vi "Vision Research Phantom Series PhFile PhNewCineFromCamera.vi"(0 "Camera Number in":u32=1, 1 "CineNr in":i32=1, 5 "Error In (no error)":errorcluster) -> (14 "Camera Number out":u32=1, 15 "CineNr out":i32, 17 "pCH":u64, 19 "Error Out":errorcluster)   [LabVIEW 2013, in "VRI.lvlib"]
doc: "PhFile.dll\n\nPhNewCineFromCamera\nHRESULT PhNewCineFromCamera(INT CN, INT CineNr, PCINEHANDLE pCH);\n\nParameters Description\nCN(in) Camera number.\nCineNr(in) Cine number. (For cameras with one cine this must be set to 1)\npCH(out) Pointer to handle of the camera cine.\nReturn HRESULT (0 = Ok)\n ERR_NOCINE – There is not any triggered cine in the camera.\nComments This function creates a cine handle that corresponds to a camera cine.\n\nWritten by:\nBLOOMY CONTROLS, INC\nWINDSOR, CT 06095, USA\n860-298-9925\nwww.bloomy.com\nV1.0.0\nMay, 2004"
uses:
  VRI.lvlib
  Phantom DLLs/PhFile.dll
panel:
  # "For instructions on the use of this VI, press Ctrl+H to display the help window and move the mouse over the icon, controls, and indicators"
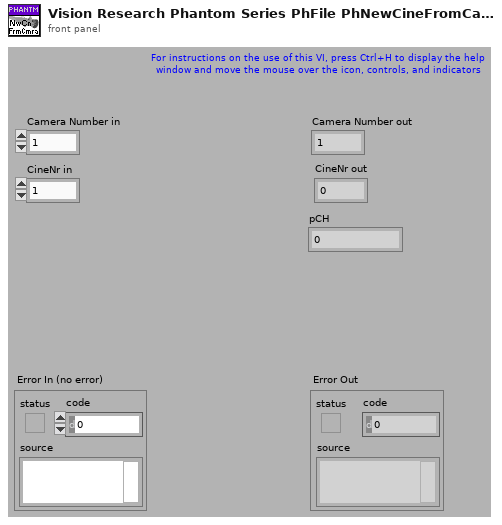
[diagram p1: front panel]
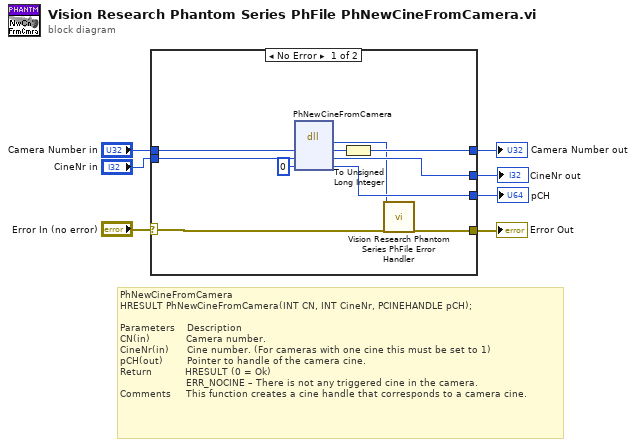
[diagram p0: block diagram]
diagram:
  # "PhNewCineFromCamera\nHRESULT PhNewCineFromCamera(INT CN, INT CineNr, PCINEHANDLE pCH);\n\nParameters    Description\nCN(in)            Camera number.\nCineNr(in)      Cine number. (For cameras with one cine this must be set to 1)\npCH(out)        Pointer to handle of the camera cine.\nReturn           HRESULT (0 = Ok)\n                      ERR_NOCINE – There is not any triggered cine in the camera.\nComments     This function creates a cine handle that corresponds to a camera cine."
  n1 = case shown="No Error" "Error In (no error)" {
    selector: "Error In (no error)" -> [w17 w20]
    tunnel: [w16 w20] -> w6
    tunnel: "Camera Number in" -> [w15 w19]
    tunnel: [w14 w19] -> w4
    tunnel: "CineNr in" -> [w13 w18]
    tunnel: [w12 _] -> w2
    tunnel: [w11 w18] -> w1
    frame No Error {
      n2 = dll-call lib="C:/Projects/SDK/32-bit/Vision Research Phantom Series Labview Driver/Phantom DLLs/PhFile.dll" fn="PhNewCineFromCamera"("CN"=w15, "CineNr"=w13, "pCH"=u64 0) -> ("HRESULT"=w9:i32, "CN"=w10:u32, "CineNr"=w11:i32, "pCH"=w12:u64)  [unwired: 3 in, 2 out]
      n3 = To Unsigned Long Integer(number=w10) -> (unsigned 32bit integer=w14:u32)
      n4 = call "Vision Research Phantom Series PhFile Error Handler.vi"("Error Code (0)"=w9, "Error In (no error)"=w17) -> ("Error Out"=w16:errorcluster)  [unwired: 17 out]
    }
    frame Error {
    }
  }
  "Error Out" <- w6
  "Camera Number out" <- w4
  "pCH" <- w2
  "CineNr out" <- w1
